vi "ZPK_change_samplingRate.vi"(10 "newSamplingTime":dbl, 11 "ZPK input cluster in":cluster{dbl, cdb[][], cdb[][], dbl}) -> (3 "Zero-Pole-Gain Model":T1 {"zero-pole-gain(s)"."delay" format="%.4f"; "zero-pole-gain(s)"."Poles" format="%#.8g"; "zero-pole-gain(s)"."Zeros" format="%#.8g"; "zero-pole-gain(s)"."Gain" format="%#.8g"; "properties"."Sampling Time" format="%#.6p"; "properties"."Output Delays" format="%.4f"; "properties"."Input Delays" format="%.4f"})   [LabVIEW 2016]
uses:
  <vilib>/addons/Control Design/_Model Construction/Model Typedefs.llb/CD Zero-Pole-Gain Model (MIMO).ctl
  <vilib>/addons/Control Design/_Model Construction/Model Typedefs.llb/CD General Elements.ctl
  <vilib>/addons/Control Design/_Model Construction/Model Typedefs.llb/CD Zero-Pole-Gain Model (SISO).ctl
  <vilib>/addons/Control Design/_Model Construction/Data Typedefs.llb/CD DtoC Conversion Method.ctl
  <vilib>/addons/Control Design/_Model Construction/Model Creation.llb/Model Creation SubVI/cd_Create Transfer Function Model.vi
  <vilib>/addons/Control Design/_Model Conversions/Model Type.llb/Model Conversion SubVI/cd_Convert Transfer Function to Zero-Pole-Gain Model.vi
  <vilib>/addons/Control Design/_Model Construction/Model Creation.llb/Model Creation SubVI/cd_Create Zero-Pole-Gain Model.vi
  <vilib>/addons/Control Design/_Model Conversions/Continuous and Discrete.llb/Continuous and Discrete SubVI/cd_Convert Discrete to Discrete (ZPK).vi
  <vilib>/addons/Control Design/_Model Interconnection/Model Interconnection.llb/Model Interconnection SubVI/cd_Matrix Multiply Models (ZPK and ZPK).vi
  <vilib>/addons/Control Design/_Model Construction/NI_LinSys_Data Typedefs.lvlib
  <vilib>/addons/Control Design/_Model Conversions/NI_CD_Continuous and Discrete.lvlib
  <vilib>/addons/Control Design/_Model Interconnection/NI_CD_Model Interconnection.lvlib
  <vilib>/addons/Control Design/_Model Construction/NI_LinSys_Model Creation.lvlib
  <vilib>/addons/Control Design/_Model Conversions/NI_CD_Model Type.lvlib
  <vilib>/addons/Control Design/_Model Construction/NI_LinSys_Model Typedefs.lvlib
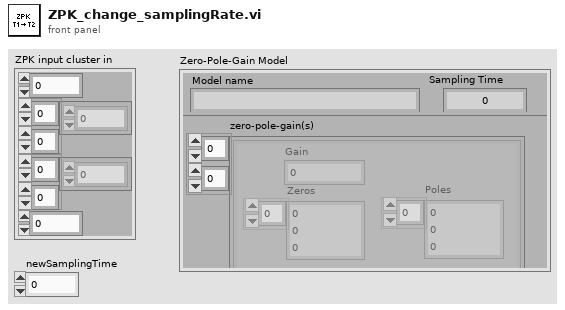
[diagram p1: front panel]
types:
  T1 = typedef "NI_LinSys_Model Typedefs.lvlib/CD Zero-Pole-Gain Model (MIMO).ctl" = cluster{"properties":T2, "zero-pole-gain(s)":T3[][]}
  T2 = typedef "NI_LinSys_Model Typedefs.lvlib/CD General Elements.ctl" = cluster{"Model name":string, "Input names":string[], "Output names":string[], "Input Delays":dbl[], "Output Delays":dbl[], "Sampling Time":dbl, "Notes":string}
  T3 = typedef "NI_LinSys_Model Typedefs.lvlib/CD Zero-Pole-Gain Model (SISO).ctl" = cluster{"Gain":dbl, "Zeros":cdb[], "Poles":cdb[], "delay":dbl}
  T4 = typedef "NI_LinSys_Model Typedefs.lvlib/CD Transfer Function Model (MIMO).ctl" = cluster{"properties":T2, "transfer function(s)":T5[][]}
  T5 = typedef "NI_LinSys_Model Typedefs.lvlib/CD Transfer Function Model (SISO).ctl" = cluster{"Numerator":dbl[], "Denominator":dbl[], "delay":dbl}
  T6 = typedef "NI_LinSys_Data Typedefs.lvlib/CD DtoC Conversion Method.ctl" = u16
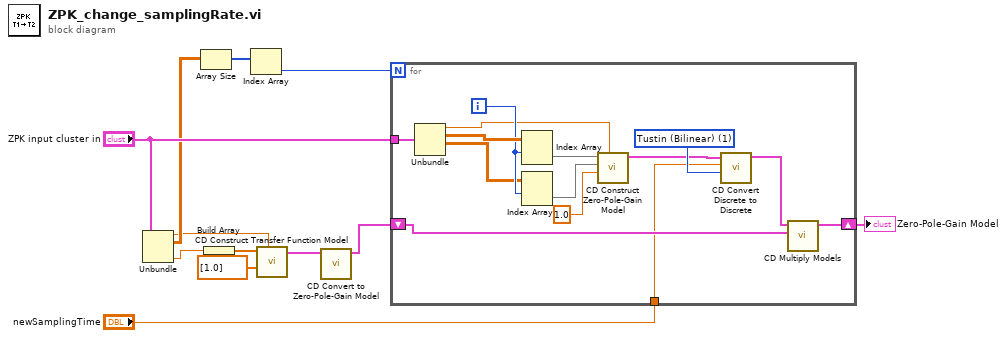
[diagram p0: block diagram]
diagram:
  n1 = Unbundle("ZPK input cluster in") -> (w1:dbl, w2:cdb[][], w9:dbl)  [unwired: 1 out]
  n2 = Array Size(array=w2) -> (size(s)=w3:i32[])
  n3 = Build Array(w9) -> (w10:dbl[])
  n4 = Index Array(array=w3) -> (element=w4:i32)  [unwired: 1 in]
  n5 = call-poly <vilib>:"CD Construct Transfer Function Model.vi"("Sampling Time (s)"=w1, "Denominator"=dbl[] [1.0], "Numerator"=w10) -> ("Transfer Function Model"=w5:T4)  [unwired: 7 in, 1 out]
  n6 = call-poly <vilib>:"CD Convert to Zero-Pole-Gain Model.vi"("Transfer Function Model"=w5) -> ("Zero-Pole-Gain Model"=w6:T1)  [unwired: 9 in, 1 out]
  n7 = for {
    N: w4 -> [_]
    tunnel: "ZPK input cluster in" -> [w13]
    shift-right: [w20] -> w7
    shift-left: w6 -> [w21]
    tunnel: "newSamplingTime" -> [w19]
    i -> [w25]
    w23 = T6 1 items=["Zero-Order-Hold", "Tustin (Bilinear)", "Prewarp", "Forward", "Backward", "Z-Transform"] ("Method")
    n8 = Unbundle(w13) -> (w14:dbl, w26:cdb[][], w24:cdb[][])  [unwired: 1 out]
    n9 = Index Array(array=w26, index (row)=w25) -> (element=w18:cdb[])  [unwired: 1 in]
    n10 = Index Array(array=w24, index (row)=w25) -> (element=w17:cdb[])  [unwired: 1 in]
    n11 = call-poly <vilib>:"CD Construct Zero-Pole-Gain Model.vi"("Sampling Time (s)"=w14, "Gain"=1.0, "Poles"=w17, "Zeros"=w18) -> ("Zero-Pole-Gain Model"=w15:T1)  [unwired: 6 in, 1 out]
    n12 = call-poly <vilib>:"CD Convert Discrete to Discrete.vi"("Method"=w23, "Resampling Time (s)"=w19, "Discrete Zero-Pole-Gain Model"=w15) -> ("Resampled Zero-Pole-Gain Model"=w22:T1)  [unwired: 7 in, 1 out]
    n13 = call-poly <vilib>:"CD Multiply Models.vi"("Model 2"=w21, "Model 1"=w22) -> ("Model Out"=w20:T1)  [unwired: 8 in, 1 out]
  }
  "Zero-Pole-Gain Model" <- w7
